vi "Set Async Status.vi"(7 "State":T1, 8 "error in (no error)":errorcluster, 11 "Status in":refnum<queue>) -> (0 "error out":errorcluster, 3 "Status out":refnum<queue>)   [LabVIEW 2020, in "SEECD Engine.lvlib"]
uses:
  SEECD Engine.lvlib
  Type Defs/Async State.ctl
  Type Defs/Async Status.ctl
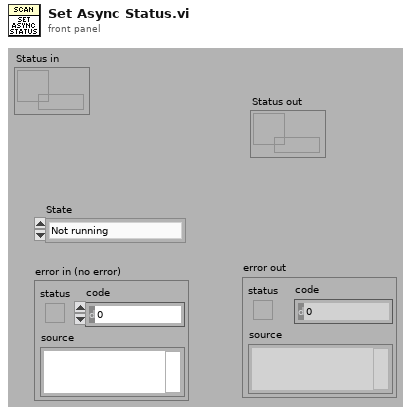
[diagram p1: front panel]
types:
  T1 = typedef "SEECD Engine.lvlib/Async State.ctl" = enum16{"Not running", "Waiting on start cmd", "Running", "Paused", "Stopped"}
  T2 = typedef "SEECD Engine.lvlib/Async Status.ctl" = cluster{"State":T1, "error":errorcluster}
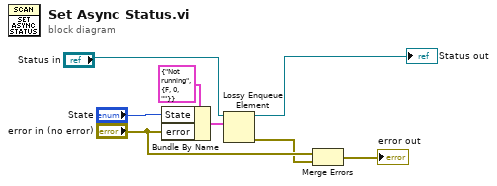
[diagram p0: block diagram]
diagram:
  n1 = Bundle By Name(cluster=T2 {"State"=enum."Not running", "error"={"status"=FALSE, "code"=0, "source"=""}} ("notification"), "State"="State", "error"="error in (no error)") -> (w8:T2)
  n2 = Lossy Enqueue Element(queue="Status in", element=w8) -> (queue out=→"Status out":refnum<queue>, error out=w2:errorcluster)  [unwired: 1 in, 2 out]
  n3 = Merge Errors("error in (no error)", w2) -> (→"error out":errorcluster)
